vi "HFRR ADV v06.vi"() -> ()   [LabVIEW 2025] (continued)
            n1807 = for {
              N: w1967 -> [_]
              tunnel: w1981 -> [w2096]
              tunnel: w1980 -> [w2095]
              tunnel: [w2085] -> w1947 mode=indexing
              tunnel: [w2083] -> w1945 mode=indexing
              tunnel: [w2084] -> w1940 mode=indexing
              tunnel: w1966 -> [_]
              tunnel: [w2077] -> w1942 mode=indexing
              tunnel: [w2073] -> w1918 mode=indexing
              tunnel: [w2069] -> w1893 mode=indexing
              tunnel: [w2065] -> w1874 mode=indexing
              tunnel: [w2060] -> w1832 mode=indexing
              (unwired) TRUE ("line mode (F)")
              n1808 = Read from Text File "Read File"(file (use dialog)=w2096, error in=w2095) -> (text=w2061:string)  [unwired: 2 in, 3 out]
              n1809 = local write "String 7"(w2061) -> ()
              n1810 = String Subset(string=w2061, offset (0)=85, length (rest)=9 ("length (rest)")) -> (substring=w2064:string)
              n1811 = String Subset(string=w2061, offset (0)=35, length (rest)=9 ("length (rest)")) -> (substring=w2086:string)
              n1812 = String Subset(string=w2061, offset (0)=55, length (rest)=9 ("length (rest)")) -> (substring=w2072:string)
              n1813 = String Subset(string=w2061, offset (0)=25, length (rest)=9 ("length (rest)")) -> (substring=w2066:string)
              n1814 = String Subset(string=w2061, offset (0)=45, length (rest)=9 ("length (rest)")) -> (substring=w2074:string)
              n1815 = String Subset(string=w2061, offset (0)=0, length (rest)=14 ("length (rest)")) -> (substring=w2089:string)
              n1816 = String Subset(string=w2061, offset (0)=15, length (rest)=9 ("length (rest)")) -> (substring=w2092:string)
              n1817 = String Subset(string=w2061, offset (0)=65, length (rest)=9 ("length (rest)")) -> (substring=w2078:string)
              n1818 = Fract/Exp String To Number(string=w2064) -> (number=w2060:dbl)  [unwired: 3 in, 1 out]
              n1819 = Fract/Exp String To Number(string=w2086) -> (number=w2084:dbl)  [unwired: 3 in, 1 out]
              n1820 = Fract/Exp String To Number(string=w2072) -> (number=w2069:dbl)  [unwired: 3 in, 1 out]
              n1821 = Fract/Exp String To Number(string=w2066) -> (number=w2065:dbl)  [unwired: 3 in, 1 out]
              n1822 = Fract/Exp String To Number(string=w2074) -> (number=w2073:dbl)  [unwired: 3 in, 1 out]
              n1823 = Fract/Exp String To Number(string=w2089) -> (number=w2085:dbl)  [unwired: 3 in, 1 out]
              n1824 = Fract/Exp String To Number(string=w2092) -> (number=w2083:dbl)  [unwired: 3 in, 1 out]
              n1825 = Fract/Exp String To Number(string=w2078) -> (number=w2081:dbl)  [unwired: 3 in, 1 out]
              n1826 = Add(x=w2081, y=0.0) -> (x+y=w2077:dbl)
            }
            n1827 = for {
              N: w1969 -> [_]
              tunnel: w1976 -> [w2024]
              tunnel: w1975 -> [w2023]
              tunnel: [w2013] -> w1929 mode=indexing
              tunnel: [w2012] -> w1922 mode=indexing
              tunnel: w1966 -> [_]
              tunnel: [w2001] -> w1927 mode=indexing
              tunnel: [w2006] -> w1924 mode=indexing
              tunnel: [w2002] -> w1914 mode=indexing
              tunnel: [w1997] -> w1889 mode=indexing
              tunnel: [w1993] -> w1870 mode=indexing
              tunnel: [w1988] -> w1830 mode=indexing
              (unwired) 1.0 ("x")
              (unwired) TRUE ("line mode (F)")
              n1828 = Read from Text File "Read File"(file (use dialog)=w2024, error in=w2023) -> (text=w1989:string)  [unwired: 2 in, 3 out]
              n1829 = local write "String 12"(w1989) -> ()
              n1830 = String Subset(string=w1989, offset (0)=85, length (rest)=9 ("length (rest)")) -> (substring=w1991:string)
              n1831 = String Subset(string=w1989, offset (0)=35, length (rest)=9 ("length (rest)")) -> (substring=w2014:string)
              n1832 = String Subset(string=w1989, offset (0)=55, length (rest)=9 ("length (rest)")) -> (substring=w1999:string)
              n1833 = String Subset(string=w1989, offset (0)=25, length (rest)=9 ("length (rest)")) -> (substring=w1995:string)
              n1834 = String Subset(string=w1989, offset (0)=45, length (rest)=9 ("length (rest)")) -> (substring=w2004:string)
              n1835 = String Subset(string=w1989, offset (0)=15, length (rest)=9 ("length (rest)")) -> (substring=w2020:string)
              n1836 = String Subset(string=w1989, offset (0)=0, length (rest)=14 ("length (rest)")) -> (substring=w2017:string)
              n1837 = String Subset(string=w1989, offset (0)=65, length (rest)=9 ("length (rest)")) -> (substring=w2007:string)
              n1838 = Fract/Exp String To Number(string=w1991) -> (number=w1988:dbl)  [unwired: 3 in, 1 out]
              n1839 = Fract/Exp String To Number(string=w2014) -> (number=w2012:dbl)  [unwired: 3 in, 1 out]
              n1840 = Fract/Exp String To Number(string=w1999) -> (number=w1997:dbl)  [unwired: 3 in, 1 out]
              n1841 = Fract/Exp String To Number(string=w1995) -> (number=w1993:dbl)  [unwired: 3 in, 1 out]
              n1842 = Fract/Exp String To Number(string=w2004) -> (number=w2002:dbl)  [unwired: 3 in, 1 out]
              n1843 = Fract/Exp String To Number(string=w2020) -> (number=w2001:dbl)  [unwired: 3 in, 1 out]
              n1844 = Fract/Exp String To Number(string=w2017) -> (number=w2013:dbl)  [unwired: 3 in, 1 out]
              n1845 = Fract/Exp String To Number(string=w2007) -> (number=w2010:dbl)  [unwired: 3 in, 1 out]
              n1846 = Add(x=w2010, y=0.0) -> (x+y=w2006:dbl)
            }
            n1847 = Delete From Array(array=w1872, index=0) -> (array with subset deleted=w1845:dbl[])  [unwired: 1 in, 1 out]
            n1848 = Delete From Array(array=w1935, index=0) -> (array with subset deleted=w1908:dbl[])  [unwired: 1 in, 1 out]
            n1849 = Delete From Array(array=w1915, index=0) -> (array with subset deleted=w1903:dbl[])  [unwired: 1 in, 1 out]
            n1850 = Delete From Array(array=w1933, index=0) -> (array with subset deleted=w1934:dbl[])  [unwired: 1 in, 1 out]
            n1851 = call-poly <vilib>:"Mean.vi"("X"=w1845) -> ("mean"=→"КОФ2 4":dbl)  [unwired: 1 out]
            n1852 = call-poly <vilib>:"Mean.vi"("X"=w1908) -> ("mean"=→"КОФ3":dbl)  [unwired: 1 out]
            n1853 = call-poly <vilib>:"Mean.vi"("X"=w1903) -> ("mean"=→"CP3":dbl)  [unwired: 1 out]
            n1854 = Delete From Array(array=w1897, index=0) -> (array with subset deleted=w1824:dbl[])  [unwired: 1 in, 1 out]
            n1855 = Delete From Array(array=w1836, index=0) -> (array with subset deleted=w1823:dbl[])  [unwired: 1 in, 1 out]
            n1856 = Delete From Array(array=w1876, index=0) -> (array with subset deleted=w1847:dbl[])  [unwired: 1 in, 1 out]
            n1857 = Delete From Array(array=w1954, index=0) -> (array with subset deleted=w1909:dbl[])  [unwired: 1 in, 1 out]
            n1858 = Delete From Array(array=w1920, index=0) -> (array with subset deleted=w1905:dbl[])  [unwired: 1 in, 1 out]
            "array w/ subset deleted" <- w1905
            n1859 = Delete From Array(array=w1951, index=0) -> (array with subset deleted=w1952:dbl[])  [unwired: 1 in, 1 out]
            n1860 = call-poly <vilib>:"Mean.vi"("X"=w1847) -> ("mean"=→"КОФ2 2":dbl)  [unwired: 1 out]
            n1861 = call-poly <vilib>:"Mean.vi"("X"=w1909) -> ("mean"=→"КОФ1":dbl)  [unwired: 1 out]
            n1862 = Bundle "Bundle"(w1824, w1823) -> (w1829:cluster{dbl[], dbl[]})  [unwired: 1 in]
            n1863 = Bundle "Bundle"(w1824, w1952) -> (w1816:cluster{dbl[], dbl[]})  [unwired: 1 in]
            n1864 = Delete From Array(array=w1831, index=0) -> (array with subset deleted=w1819:dbl[])  [unwired: 1 in, 1 out]
            n1865 = Delete From Array(array=w1832, index=0) -> (array with subset deleted=w1821:dbl[])  [unwired: 1 in, 1 out]
            n1866 = Delete From Array(array=w1942, index=0) -> (array with subset deleted=w1943:dbl[])  [unwired: 1 in, 1 out]
            n1867 = Delete From Array(array=w1830, index=0) -> (array with subset deleted=w1817:dbl[])  [unwired: 1 in, 1 out]
            n1868 = Delete From Array(array=w1924, index=0) -> (array with subset deleted=w1925:dbl[])  [unwired: 1 in, 1 out]
            n1869 = Delete From Array(array=w1949, index=0) -> (array with subset deleted=w1855:dbl[])  [unwired: 1 in, 1 out]
            n1870 = Delete From Array(array=w1895, index=0) -> (array with subset deleted=w1851:dbl[])  [unwired: 1 in, 1 out]
            n1871 = Delete From Array(array=w1931, index=0) -> (array with subset deleted=w1853:dbl[])  [unwired: 1 in, 1 out]
            n1872 = Delete From Array(array=w1891, index=0) -> (array with subset deleted=w1849:dbl[])  [unwired: 1 in, 1 out]
            n1873 = Delete From Array(array=w1940, index=0) -> (array with subset deleted=w1854:dbl[])  [unwired: 1 in, 1 out]
            n1874 = Delete From Array(array=w1893, index=0) -> (array with subset deleted=w1850:dbl[])  [unwired: 1 in, 1 out]
            n1875 = Delete From Array(array=w1874, index=0) -> (array with subset deleted=w1846:dbl[])  [unwired: 1 in, 1 out]
            n1876 = Delete From Array(array=w1918, index=0) -> (array with subset deleted=w1904:dbl[])  [unwired: 1 in, 1 out]
            n1877 = Delete From Array(array=w1945, index=0) -> (array with subset deleted=w1906:dbl[])  [unwired: 1 in, 1 out]
            n1878 = Delete From Array(array=w1922, index=0) -> (array with subset deleted=w1852:dbl[])  [unwired: 1 in, 1 out]
            n1879 = Delete From Array(array=w1889, index=0) -> (array with subset deleted=w1848:dbl[])  [unwired: 1 in, 1 out]
            n1880 = Delete From Array(array=w1870, index=0) -> (array with subset deleted=w1844:dbl[])  [unwired: 1 in, 1 out]
            n1881 = Delete From Array(array=w1914, index=0) -> (array with subset deleted=w1902:dbl[])  [unwired: 1 in, 1 out]
            n1882 = Delete From Array(array=w1927, index=0) -> (array with subset deleted=w1907:dbl[])  [unwired: 1 in, 1 out]
            n1883 = Delete From Array(array=w1937, index=0) -> (array with subset deleted=w1820:dbl[])  [unwired: 1 in, 1 out]
            n1884 = Delete From Array(array=w1947, index=0) -> (array with subset deleted=w1822:dbl[])  [unwired: 1 in, 1 out]
            n1885 = Delete From Array(array=w1929, index=0) -> (array with subset deleted=w1818:dbl[])  [unwired: 1 in, 1 out]
            n1886 = Bundle "Bundle"(w1824, w1855) -> (w1842:cluster{dbl[], dbl[]})  [unwired: 1 in]
            n1887 = Bundle "Bundle"(w1824, w1909) -> (w1843:cluster{dbl[], dbl[]})  [unwired: 1 in]
            n1888 = Bundle "Bundle"(w1855, w1851) -> (w1857:cluster{dbl[], dbl[]})  [unwired: 1 in]
            n1889 = Bundle "Bundle"(w1820, w1819) -> (w1827:cluster{dbl[], dbl[]})  [unwired: 1 in]
            n1890 = Bundle "Bundle"(w1853, w1849) -> (w1859:cluster{dbl[], dbl[]})  [unwired: 1 in]
            n1891 = Bundle "Bundle"(w1820, w1853) -> (w1963:cluster{dbl[], dbl[]})  [unwired: 1 in]
            n1892 = Bundle "Bundle"(w1820, w1849) -> (w1887:cluster{dbl[], dbl[]})  [unwired: 1 in]
            n1893 = Bundle "Bundle"(w1820, w1908) -> (w1973:cluster{dbl[], dbl[]})  [unwired: 1 in]
            n1894 = Bundle "Bundle"(w1820, w1903) -> (w1911:cluster{dbl[], dbl[]})  [unwired: 1 in]
            n1895 = Bundle "Bundle"(w1820, w1934) -> (w1958:cluster{dbl[], dbl[]})  [unwired: 1 in]
            n1896 = Bundle "Bundle"(w1854, w1850) -> (w1858:cluster{dbl[], dbl[]})  [unwired: 1 in]
            n1897 = Bundle "Bundle"(w1822, w1821) -> (w1828:cluster{dbl[], dbl[]})  [unwired: 1 in]
            n1898 = Bundle "Bundle"(w1822, w1854) -> (w1965:cluster{dbl[], dbl[]})  [unwired: 1 in]
            n1899 = Bundle "Bundle"(w1822, w1850) -> (w1888:cluster{dbl[], dbl[]})  [unwired: 1 in]
            n1900 = Bundle "Bundle"(w1822, w1904) -> (w1912:cluster{dbl[], dbl[]})  [unwired: 1 in]
            n1901 = Bundle "Bundle"(w1822, w1906) -> (w1974:cluster{dbl[], dbl[]})  [unwired: 1 in]
            n1902 = Bundle "Bundle"(w1822, w1943) -> (w1956:cluster{dbl[], dbl[]})  [unwired: 1 in]
            n1903 = Bundle "Bundle"(w1852, w1848) -> (w1860:cluster{dbl[], dbl[]})  [unwired: 1 in]
            n1904 = Bundle "Bundle"(w1818, w1817) -> (w1826:cluster{dbl[], dbl[]})  [unwired: 1 in]
            n1905 = Bundle "Bundle"(w1818, w1852) -> (w1964:cluster{dbl[], dbl[]})  [unwired: 1 in]
            n1906 = Bundle "Bundle"(w1818, w1848) -> (w1886:cluster{dbl[], dbl[]})  [unwired: 1 in]
            n1907 = Bundle "Bundle"(w1818, w1902) -> (w1910:cluster{dbl[], dbl[]})  [unwired: 1 in]
            n1908 = Bundle "Bundle"(w1818, w1907) -> (w1972:cluster{dbl[], dbl[]})  [unwired: 1 in]
            n1909 = Bundle "Bundle"(w1818, w1925) -> (w1957:cluster{dbl[], dbl[]})  [unwired: 1 in]
            n1910 = call-poly <vilib>:"Mean.vi"("X"=w1905) -> ("mean"=→"CP1":dbl)  [unwired: 1 out]
            n1911 = call-poly <vilib>:"Mean.vi"("X"=w1846) -> ("mean"=→"КОФ2 3":dbl)  [unwired: 1 out]
            n1912 = call-poly <vilib>:"Mean.vi"("X"=w1904) -> ("mean"=→"CP2":dbl)  [unwired: 1 out]
            n1913 = call-poly <vilib>:"Mean.vi"("X"=w1906) -> ("mean"=→"КОФ2":dbl)  [unwired: 1 out]
            n1914 = call-poly <vilib>:"Mean.vi"("X"=w1844) -> ("mean"=→"КОФ2 5":dbl)  [unwired: 1 out]
            n1915 = call-poly <vilib>:"Mean.vi"("X"=w1902) -> ("mean"=→"CP4":dbl)  [unwired: 1 out]
            n1916 = call-poly <vilib>:"Mean.vi"("X"=w1907) -> ("mean"=→"КОФ4":dbl)  [unwired: 1 out]
            n1917 = Bundle "Bundle"(w1824, w1851) -> (w1815:cluster{dbl[], dbl[]})  [unwired: 1 in]
            n1918 = Bundle "Bundle"(w1824, w1905) -> (w1838:cluster{dbl[], dbl[]})  [unwired: 1 in]
            n1919 = Build Array "Build Array"(w1815, w1838) -> (w1841:cluster{dbl[], dbl[]}[])
            "XY Graph 17" <- w1841
            n1920 = Build Array "Build Array"(w1829, w1828, w1827, w1826) -> (→"Frequency ( Hz )":cluster{dbl[], dbl[]}[])
            n1921 = Build Array "Build Array"(w1857, w1858, w1859, w1860) -> (→"Air Temp ( °C ) vs Humidity ( % RH )":cluster{dbl[], dbl[]}[])
            n1922 = Build Array "Build Array"(w1842, w1965, w1963, w1964) -> (→"Air Temperature  ( °C )":cluster{dbl[], dbl[]}[])
            n1923 = Build Array "Build Array"(w1815, w1888, w1887, w1886) -> (→"Humidity ( %RH )":cluster{dbl[], dbl[]}[])
            n1924 = Build Array "Build Array"(w1843, w1974, w1973, w1972) -> (→"Coefficient Of Friction":cluster{dbl[], dbl[]}[])
            n1925 = Build Array "Build Array"(w1838, w1912, w1911, w1910) -> (→"Sample Temperature ( °C )":cluster{dbl[], dbl[]}[])
            n1926 = Build Array "Build Array"(w1816, w1956, w1958, w1957) -> (→"XY Graph 13":cluster{dbl[], dbl[]}[])
            n1927 = Bundle "Bundle"(w1824, w1847) -> (w1869:cluster{dbl[], dbl[]})  [unwired: 1 in]
            n1928 = Bundle "Bundle"(w1820, w1845) -> (w1867:cluster{dbl[], dbl[]})  [unwired: 1 in]
            n1929 = Bundle "Bundle"(w1822, w1846) -> (w1868:cluster{dbl[], dbl[]})  [unwired: 1 in]
            n1930 = Bundle "Bundle"(w1818, w1844) -> (w1866:cluster{dbl[], dbl[]})  [unwired: 1 in]
            n1931 = Build Array "Build Array"(w1869, w1868, w1867, w1866) -> (→"Stroke ( mm )":cluster{dbl[], dbl[]}[])
            n1932 = local write "XY Graph 16"(w1841) -> ()
          }
          frame #2 {
          }
          frame #3 {
            n1933 = local write "Numeric 8"(0 ("Numeric 8")) -> ()
            n1934 = local write "Numeric 11"(0 ("Numeric 11")) -> ()
            n1935 = local write "Numeric 12"(0 ("Numeric 12")) -> ()
            n1936 = local write "Numeric 13"(0 ("Numeric 13")) -> ()
            n1937 = property on="OPEN" class="Bool (strict)"("Visible"=TRUE) -> ()  [unwired: 2 in, 2 out]
            n1938 = local read "String Control 2"() -> (w2141:string)
            n1939 = local read "String Control 4"() -> (w2140:string)
            n1940 = local read "String Control 6"() -> (w2139:string)
            n1941 = local read "String Control 8"() -> (w2138:string)
            n1942 = Match Pattern(string=w2141, regular expression="Samples / cycle :- ") -> (after substring=w2155:string)  [unwired: 1 in, 3 out]
            n1943 = Match Pattern(string=w2141, regular expression="Frequency :- ") -> (after substring=w2174:string)  [unwired: 1 in, 3 out]
            n1944 = Match Pattern(string=w2140, regular expression="Samples / cycle :- ") -> (after substring=w2151:string)  [unwired: 1 in, 3 out]
            n1945 = Match Pattern(string=w2140, regular expression="Frequency :- ") -> (after substring=w2169:string)  [unwired: 1 in, 3 out]
            n1946 = Match Pattern(string=w2139, regular expression="Samples / cycle :- ") -> (after substring=w2147:string)  [unwired: 1 in, 3 out]
            n1947 = Match Pattern(string=w2139, regular expression="Frequency :- ") -> (after substring=w2164:string)  [unwired: 1 in, 3 out]
            n1948 = Match Pattern(string=w2138, regular expression="Samples / cycle :- ") -> (after substring=w2143:string)  [unwired: 1 in, 3 out]
            n1949 = Match Pattern(string=w2138, regular expression="Frequency :- ") -> (after substring=w2159:string)  [unwired: 1 in, 3 out]
            n1950 = String Subset(string=w2155, length (rest)=6 ("length (rest)")) -> (substring=w2157:string)  [unwired: 1 in]
            n1951 = String Subset(string=w2174, length (rest)=9 ("length (rest)")) -> (substring=w2176:string)  [unwired: 1 in]
            n1952 = String Subset(string=w2151, length (rest)=6 ("length (rest)")) -> (substring=w2153:string)  [unwired: 1 in]
            n1953 = String Subset(string=w2169, length (rest)=9 ("length (rest)")) -> (substring=w2171:string)  [unwired: 1 in]
            n1954 = String Subset(string=w2147, length (rest)=6 ("length (rest)")) -> (substring=w2149:string)  [unwired: 1 in]
            n1955 = String Subset(string=w2164, length (rest)=9 ("length (rest)")) -> (substring=w2166:string)  [unwired: 1 in]
            n1956 = String Subset(string=w2143, length (rest)=6 ("length (rest)")) -> (substring=w2145:string)  [unwired: 1 in]
            n1957 = String Subset(string=w2159, length (rest)=9 ("length (rest)")) -> (substring=w2161:string)  [unwired: 1 in]
            n1958 = Fract/Exp String To Number(string=w2157) -> (number=w2137:dbl)  [unwired: 3 in, 1 out]
            n1959 = Fract/Exp String To Number(string=w2176) -> (number=w2177:dbl)  [unwired: 3 in, 1 out]
            n1960 = Fract/Exp String To Number(string=w2153) -> (number=w2136:dbl)  [unwired: 3 in, 1 out]
            n1961 = Fract/Exp String To Number(string=w2171) -> (number=w2172:dbl)  [unwired: 3 in, 1 out]
            n1962 = Fract/Exp String To Number(string=w2149) -> (number=w2135:dbl)  [unwired: 3 in, 1 out]
            n1963 = Fract/Exp String To Number(string=w2166) -> (number=w2167:dbl)  [unwired: 3 in, 1 out]
            n1964 = Fract/Exp String To Number(string=w2145) -> (number=w2134:dbl)  [unwired: 3 in, 1 out]
            n1965 = Fract/Exp String To Number(string=w2161) -> (number=w2162:dbl)  [unwired: 3 in, 1 out]
            n1966 = local write "sample1"(w2137) -> ()
            n1967 = local write "freq1"(w2177) -> ()
            n1968 = local write "sample2"(w2136) -> ()
            n1969 = local write "freq2"(w2172) -> ()
            n1970 = local write "sample3"(w2135) -> ()
            n1971 = local write "freq3"(w2167) -> ()
            n1972 = local write "sample4"(w2134) -> ()
            n1973 = local write "freq 4"(w2162) -> ()
          }
        }
      }
    }
    n1974 = case shown="True" w1626 {
      selector: w1626 -> [_ w1754]
      frame False {
      }
      frame True {
        n1975 = Not(x=w1754) -> (.not. x?=w1750:bool)
        n1976 = local write "service 3"(w1750) -> ()
        n1977 = local write "OPEN 6"(w1750) -> ()
        n1978 = call <vilib>:"System Exec.vi"("wait until completion? (T)"=TRUE, "command line"="C:\\LAB-IQ\\Scar View.exe") -> ("error out"=→"error out 5":errorcluster)  [unwired: 6 in, 3 out]
      }
    }
    n1979 = case shown="\"Acquire\", Default" w1637 {
      frame "Acquire", Default {
        w2650 = 0.2 ("y")
        w2655 = 1.0 ("y")
        w2656 = 0.8 ("y")
        # "Elapsed time\ncof\nstroke\nAir temp\nTemp\nHumidity"
        n1980 = disable-structure shown="Disabled" {
          frame Disabled {
            n1981 = local read "Flag"() -> (w2673:dbl)
            n1982 = local read "RUN"() -> (w2670:bool)
            n1983 = Not(x=w2670) -> (.not. x?=w2669:bool)
            n1984 = Equal?(x=w2673, y=10.0) -> (x = y?=w2671:bool)
            n1985 = And(x=w2671, y=w2669) -> (x .and. y?=w2668:bool)
            n1986 = case shown="True" w2668 {
              frame False {
              }
              frame True {
                w2674 = FALSE ("Heater Button")
                n1987 = local write "Humidity"(w2674) -> ()
                n1988 = local write "Heater Button"(w2674) -> ()
              }
            }
          }
          frame Enabled {
          }
        }
        n1989 = disable-structure shown="Disabled" {
          frame Disabled {
            n1990 = case shown="True" {
              selector: _ -> [_ _]
              frame False {
              }
              frame True {
                w2765 = TRUE ("Heater")
                n1991 = local write "Humidity"(w2765) -> ()
                n1992 = local write "Heater Button"(w2765) -> ()
                n1993 = local read "TEST STANDARD"() -> (w2768:T3)
                n1994 = local read "TEST STANDARD"() -> (w2763:T3)
                n1995 = Equal?(x=w2768, y=enum16{"ASTM D6079", "ISO 12156", "Custom"}."ISO 12156" ("Test Standard")) -> (x = y?=w2766:bool)
                n1996 = Equal?(x=w2763, y=enum16{"ASTM D6079", "ISO 12156", "Custom"}."ASTM D6079" ("Test Standard")) -> (x = y?=w2762:bool)
                n1997 = case shown="True" w2766 {
                  frame False {
                  }
                  frame True {
                    n1998 = local write "Heater"(TRUE ("Heater")) -> ()
                    n1999 = local write "airtempflg"(FALSE ("airtempflg")) -> ()
                  }
                }
                n2000 = case shown="True" w2762 {
                  frame False {
                  }
                  frame True {
                    n2001 = local write "Heater"(FALSE ("Heater")) -> ()
                    n2002 = local write "airtempflg"(TRUE ("airtempflg")) -> ()
                  }
                }
              }
            }
          }
          frame Enabled {
          }
        }
        n2003 = stacked-sequence {
          frame #0 {
            n2004 = case shown="True" "RST FF" {
              frame False {
              }
              frame True {
                w2831 = 0.0 ("X Scale.Range:Maximum")
                n2005 = property on="Frictional Force ( N )" class="WFChart (strict)"("XScale.Maximum"=600.0 ("X Scale.Range:Maximum"), "XScale.Minimum"=w2831, "YScale.Maximum"=10.0 ("Y Scale.Range:Maximum"), "YScale.Minimum"=w2831) -> ()  [unwired: 2 in, 2 out]
              }
            }
          }
          frame #1 {
            n2006 = case shown="True" "RST TEMP" {
              frame False {
              }
              frame True {
                n2007 = property on="Temperature ( Deg C )" class="WFChart (strict)"("XScale.Minimum"=0.0 ("X Scale.Range:Minimum"), "XScale.Maximum"=600.0 ("X Scale.Range:Maximum"), "YScale.Minimum"=0.0 ("Y Scale.Range:Minimum"), "YScale.Maximum"=100.0 ("Y Scale.Range:Maximum")) -> ()  [unwired: 2 in, 2 out]
              }
            }
          }
          frame #2 {
            n2008 = case shown="True" "RSTCOF" {
              frame False {
              }
              frame True {
                n2009 = property on="Coefficient of Friction" class="WFChart (strict)"("XScale.Minimum"=0.0 ("X Scale.Range:Minimum"), "XScale.Maximum"=600.0 ("X Scale.Range:Maximum"), "YScale.Maximum"=1.0 ("X Scale.Range:Minimum"), "YScale.Minimum"=0.0 ("X Scale.Range:Minimum")) -> ()  [unwired: 2 in, 2 out]
              }
            }
          }
          frame #3 {
            n2010 = case shown="True" "RSTCOF 2" {
              frame False {
              }
              frame True {
                (unwired) 100.0 ("Y Scale.Range:Maximum")
                (unwired) 0.0 ("Y Scale.Range:Minimum")
                (unwired) 600.0 ("X Scale.Range:Maximum")
                (unwired) 0.0 ("X Scale.Range:Minimum")
              }
            }
          }
          frame #4 {
            n2011 = case shown="True" "RSTCOF 3" {
              frame False {
              }
              frame True {
                n2012 = property on="Electrical Contact Resistance ( % )" class="WFChart (strict)"("XScale.Minimum"=0.0 ("X Scale.Range:Minimum"), "XScale.Maximum"=600.0 ("X Scale.Range:Maximum"), "YScale.Minimum"=0.0 ("Y Scale.Range:Minimum"), "YScale.Maximum"=100.0 ("Y Scale.Range:Maximum")) -> ()  [unwired: 2 in, 2 out]
              }
            }
          }
        }
        n2013 = disable-structure shown="Disabled" {
          frame Disabled {
            n2014 = case shown="True" {
              selector: _ -> [_ _]
              frame False {
              }
              frame True {
                n2015 = local read "zflag 2"() -> (w2732:dbl)
                n2016 = local read "yflag"() -> (w2734:dbl)
                n2017 = Equal?(x=w2734, y=2.0 ("tflag")) -> (x = y?=w2736:bool)
                n2018 = Equal?(x=w2732, y=3.0 ("tflag")) -> (x = y?=w2735:bool)
                n2019 = And(x=w2736, y=w2735) -> (x .and. y?=w2730:bool)
                n2020 = case shown="True" w2730 {
                  frame False {
                  }
                  frame True {
                    w2761 = 0.0 ("zflag")
                    n2021 = local write "zflag"(w2761) -> ()
                    n2022 = local write "zflag 2"(w2761) -> ()
                    n2023 = Delete(path (use dialog)=path "C:/LAB-IQ-NXT/WO 2449 TT.sig" ("file path (dialog if empty)")) -> (deleted path=w2760:path)  [unwired: 4 in, 2 out]
                    n2024 = Delete(path (use dialog)=path "C:/LAB-IQ-NXT/WO 2449 TRH.sig" ("file path (dialog if empty)")) -> (deleted path=w2755:path)  [unwired: 4 in, 2 out]
                    n2025 = local read "SEN.RUN HRS"() -> (w2747:dbl)
                    n2026 = local read "SENSOR TIME"() -> (w2745:dbl)
                    n2027 = call <vilib>:"compatOverwrite.vi"("overwrite (F)"=TRUE) -> ("overwrite?"=w2737:T27)
                    n2028 = call <vilib>:"compatOverwrite.vi"("overwrite (F)"=TRUE) -> ("overwrite?"=w2741:T27)
                    n2029 = local read "Total No. of Tests"() -> (w2748:dbl)
                    n2030 = Add(x=w2745, y=w2747) -> (x+y=w2746:dbl)
                    "SEN.RUN HRS" <- w2746
                    n2031 = Open/Create/Replace File(file path (use dialog)=w2760, operation (0:open)=w2737) -> (refnum out=w2738:refnum<file>, error out=w2739:errorcluster)  [unwired: 4 in, 1 out]
                    n2032 = Open/Create/Replace File(file path (use dialog)=w2755, operation (0:open)=w2741) -> (refnum out=w2742:refnum<file>, error out=w2743:errorcluster)  [unwired: 4 in, 1 out]
                    n2033 = Deny Access(4:w2739, 6:T24."deny none" ("deny mode (2)"), 7:w2738) -> (3:w2759:refnum<file>)  [unwired: 1 out]
                    n2034 = Deny Access(4:w2743, 6:T24."deny none" ("deny mode (2)"), 7:w2742) -> (3:w2751:refnum<file>)  [unwired: 1 out]
                    n2035 = Number To Decimal String(number=w2748) -> (decimal integer string=w2756:string)  [unwired: 1 in]
                    n2036 = Number To Decimal String(number=w2746) -> (decimal integer string=w2752:string)  [unwired: 1 in]
                    n2037 = Write to Binary File(file (use dialog)=w2759, data=w2756, 5:FALSE ("prepend array or string size? (T)")) -> ()  [unwired: 3 in, 3 out]
                    n2038 = Write to Binary File(file (use dialog)=w2751, data=w2752, 5:FALSE ("prepend array or string size? (T)")) -> ()  [unwired: 3 in, 3 out]
                  }
                }
              }
            }
          }
          frame Enabled {
          }
        }
        n2039 = local read "RUN"() -> (w2659:bool)
        n2040 = local read "run replace"() -> (w2663:bool)
        n2041 = local read "run replace"() -> (w2662:bool)
        n2042 = case shown="True" w2659 {
          frame False {
            n2043 = local write "run replace"(FALSE ("run replace")) -> ()
          }
          frame True {
            "run replace" <- TRUE ("run replace")
          }
        }
        n2044 = local read "RUN"() -> (w2667:bool)
        n2045 = local read "Set Temp"() -> (w2629:dbl)
        n2046 = local read "SetTemp"() -> (w2631:dbl)
        n2047 = case shown="False" w2667 {
          tunnel: [FALSE ("TEST RUNNING") TRUE ("TEST RUNNING")] -> w2666
          frame False {
            w2850 = 0.0 ("Flag")
            n2048 = local write "Elapsed time"(0.0 ("elapsedtime")) -> ()
            n2049 = local write "Time Remaining"(w2850) -> ()
            n2050 = local write "Flag"(w2850) -> ()
            n2051 = local write "Remaining Time"(w2850) -> ()
          }
          frame True {
            n2052 = local write "Flag"(10.0 ("Flag")) -> ()
          }
        }
        n2053 = case shown="False" w2663 {
          frame False {
            n2054 = local read "zflag"() -> (→"zflag 2":dbl)
            n2055 = local write "yflag"(2.0 ("tflag")) -> ()
            n2056 = local write "FLAG 4"(0.0 ("FLAG")) -> ()
          }
          frame True {
            n2057 = local write "yflag"(1.0 ("tflag")) -> ()
            n2058 = local write "zflag"(3.0 ("zflag")) -> ()
          }
        }
        n2059 = local read "acq 2"() -> (w2661:bool)
        n2060 = local read "AIR TEMP"() -> (w2624:dbl)
        n2061 = local read "Amb temp"() -> (w2628:dbl)
        n2062 = case shown="True" "Save & Continue" {
          frame False {
          }
          frame True {
            "acq 2" <- TRUE ("acq 2")
          }
        }
        n2063 = local read "Set Rh"() -> (w2630:dbl)
        n2064 = Add(x=w2631, y=w2656) -> (x+y=w2657:dbl)
        n2065 = Subtract(x=w2631, y=w2656) -> (x-y=w2658:dbl)
        n2066 = Add(x=w2629, y=w2650) -> (x+y=w2651:dbl)
        n2067 = Subtract(x=w2629, y=w2650) -> (x-y=w2652:dbl)
        n2068 = And(x=w2661, y=w2662) -> (x .and. y?=w2660:bool)
        n2069 = Greater Or Equal?(x=w2624, y=15.0) -> (x >= y?=w2625:bool)
        "powstat" <- w2625
        n2070 = local read "Humidity ( %RH )"() -> (w2627:dbl)
        n2071 = case shown="True" "Save & Continue" {
          frame False {
          }
          frame True {
            n2072 = while {
              tunnel: "0123456789abcdefghijklmnopqrstuvwxyzABCDEFGHIJKLMNOPQRSTUVWXYZ" ("string 2") -> [w2821]
              shift-right: [w2819] -> w2814
              shift-left: "" -> [w2818]
              i -> [w2828]
              stop <- w2827 stop-if-true
              n2073 = Random Number (0-1)() -> (number: 0 to 1=w2822:dbl)
              n2074 = Multiply(x=w2822, y=62.0) -> (x*y=w2824:dbl)
              n2075 = Decrement(x="Length") -> (x-1=w2817:i16)
              n2076 = To Word Integer(number=w2824) -> (16bit integer=w2825:i16)
              n2077 = String Subset(string=w2821, offset (0)=w2825, length (rest)=1 ("length (rest)")) -> (substring=w2820:string)
              n2078 = Greater Or Equal?(x=w2828, y=w2817) -> (x >= y?=w2827:bool)
              n2079 = Concatenate Strings(w2820, w2818) -> (w2819:string)
            }
            n2080 = local write "UUID"(w2814) -> ()
          }
        }
        n2081 = In Range and Coerce(upper limit=w2657, x=w2628, lower limit=w2658) -> (In Range?=w2647:bool)  [unwired: 1 out]
        n2082 = Add(x=w2630, y=w2655) -> (x+y=w2654:dbl)
        n2083 = Subtract(x=w2630, y=w2655) -> (x-y=w2653:dbl)
        n2084 = local read "TEMP"() -> (w2626:dbl)
        n2085 = case shown="True" "Save & Continue" {
          frame False {
          }
          frame True {
            n2086 = local read "Operator ID"() -> (w3130:string)
            n2087 = local read "FILE"() -> (w3136:string)
            n2088 = String Length(string=w3136) -> (length=w3134:i32)
            n2089 = String Length(string=w3130) -> (length=w3131:i32)
            n2090 = Greater?(x=w3134, y=0) -> (0:w3133:bool)
            n2091 = Greater?(x=w3131, y=0) -> (0:w3129:bool)
            n2092 = And(x=w3133, y=w3129) -> (x .and. y?=w3128:bool)
            n2093 = case shown="True" w3128 {
              frame False {
                n2094 = stacked-sequence {
                  frame #0 {
                    n2095 = One Button Dialog(message="Please Enter a File Name and Operator ID to save data !", button name ("OK")="Ok") -> ()  [unwired: 1 out]
                  }
                  frame #1 {
                    n2096 = local write "Save & Continue"(FALSE ("OK Button")) -> ()
                  }
                }
                n2097 = local write "Save & Continue"(FALSE ("OK Button")) -> ()
              }
              frame True {
                n2098 = stacked-sequence {
                  frame #0 {
                    n2099 = local read "FILE"() -> (w3142:string)
                    n2100 = call "file check.vi"("file name in"=w3142) -> ("file name out"=w3141:string)  [unwired: 9 in, 1 out]
                    n2101 = call <vilib>:"Application Directory.vi"() -> ("Application Directory"=w3152:path)
                    n2102 = Build Path(base path=w3152, name or relative path="data") -> (appended path=w3151:path)
                    n2103 = call <vilib>:"Trim Whitespace.vi"("string"=w3141) -> ("trimmed string"=w3149:string)  [unwired: 1 in]
                    n2104 = call <vilib>:"Trim Whitespace.vi"("string"=w3141) -> ("trimmed string"=w3150:string)  [unwired: 1 in]
                    n2105 = List Folder(path=w3151) -> (folder names=w3147:string[])  [unwired: 3 in, 3 out]
                    n2106 = Match Pattern(string=w3149, regular expression="_(") -> (before substring=w3146:string)  [unwired: 1 in, 3 out]
                    n2107 = for {
                      tunnel: w3147 -> [w3161] mode=indexing
                      tunnel: w3146 -> [w3159]
                      shift-right: [w3157] -> w3144
                      shift-left: bool[] [] -> [w3158]
                      n2108 = Match Pattern(string=w3161, regular expression="_(") -> (before substring=w3160:string)  [unwired: 1 in, 3 out]
                      n2109 = Equal?(x=w3160, y=w3159) -> (x = y?=w3156:bool)
                      n2110 = case shown="True" w3156 {
                        tunnel: w3156 -> [_ w3164]
                        tunnel: w3158 -> [w3163 w3166]
                        tunnel: [w3163 w3165] -> w3157
                        frame False {
                        }
                        frame True {
                          n2111 = Insert Into Array(array=w3166, new element=w3164) -> (w3165:bool[])  [unwired: 1 in]
                        }
                      }
                    }
                    n2112 = Equal?(x=w3147, y=w3146) -> (x = y?=w3155:bool[])
                    n2113 = Or Array Elements(Boolean array=w3155) -> (logical OR=w3154:bool)
                    n2114 = Array Size(array=w3144) -> (size(s)=w3143:i32)
                    n2115 = case shown="True" w3154 {
                      tunnel: w3150 -> [_ w3174]
                      tunnel: w3143 -> [_ w3167]
                      frame False {
                      }
                      frame True {
                        n2116 = Number To Decimal String(number=w3167) -> (decimal integer string=w3170:string)  [unwired: 1 in]
                        n2117 = Search/Split String(string=w3174, search string/char (-)="_(" ("regular expression")) -> (substring before match=w3172:string)  [unwired: 1 in, 2 out]
                        n2118 = Concatenate Strings(w3172, "_(" ("regular expression"), w3170, ")" ("regular expression")) -> (w3168:string)
                        n2119 = local write "FILE"(w3168) -> ()
                      }
                    }
                  }
                  frame #1 {
                    w3176 = 0.0
                    w3189 = cluster{"y":dbl, dbl, "y":dbl}[] [] ("History Data")
                    w3190 = FALSE ("Heater Button")
                    (unwired) ")!" ("string")
                    (unwired) ")" ("string")
                    w3188 = dbl[] [] ("History Data")
                    w3194 = "\r"
                    # "C:\\WinDucom\\Data\\"
                    # "C:\\LAB-IQ-NXT\\data"
                    n2120 = local write "Humidity ( %RH )"(w3176) -> ()
                    n2121 = local write "Frequency ( Hz )"(w3176) -> ()
                    n2122 = local write "Stroke 3"(w3176) -> ()
                    n2123 = local write "speedop"(0.0 ("PIDclk 2")) -> ()
                    n2124 = local write "Set Temp 2"(65.0 ("Set Temp 2")) -> ()
                    n2125 = local write "AIR TEMP"(w3176) -> ()
                    n2126 = local write "clk"(0.0 ("clk")) -> ()
                    n2127 = local write "Stroke 4"(w3176) -> ()
                    n2128 = local write "COF 2"(w3176) -> ()
                    n2129 = local write "TEMP"(w3176) -> ()
                    n2130 = local write "ecr 3"(w3176) -> ()
                    n2131 = local write "FF 3"(w3176) -> ()
                    n2132 = local write "FF 2"(w3176) -> ()
                    n2133 = property on="Humidity ( %RH )" class="WFChart (strict)"("History Data"=w3188) -> ()  [unwired: 2 in, 2 out]
                    n2134 = property on="Coefficient of Friction" class="WFChart (strict)"("History Data"=w3188) -> ()  [unwired: 2 in, 2 out]
                    n2135 = property on="Coefficient of Friction" class="WFChart (strict)"("History Data"=w3188) -> ()  [unwired: 2 in, 2 out]
                    n2136 = property on="Frictional Force ( N )" class="WFChart (strict)"("History Data"=w3188) -> ()  [unwired: 2 in, 2 out]
                    n2137 = property on="Electrical Contact Resistance ( % )" class="WFChart (strict)"("History Data"=w3188) -> ()  [unwired: 2 in, 2 out]
                    n2138 = property on="Electrical Contact Resistance ( % )" class="WFChart (strict)"("History Data"=w3188) -> ()  [unwired: 2 in, 2 out]
                    n2139 = property on="Temperature ( Deg C )" class="WFChart (strict)"("History Data"=w3188) -> ()  [unwired: 2 in, 2 out]
                    n2140 = property on="Frictional Force ( N )" class="WFChart (strict)"("History Data"=w3188) -> ()  [unwired: 2 in, 2 out]
                    n2141 = property on="Coefficient of Friction" class="WFChart (strict)"("History Data"=w3188) -> ()  [unwired: 2 in, 2 out]
                    n2142 = property on="Frictional Force ( N )" class="WFChart (strict)"("History Data"=w3188) -> ()  [unwired: 2 in, 2 out]
                    n2143 = property on="Electrical Contact Resistance ( % )" class="WFChart (strict)"("History Data"=w3188) -> ()  [unwired: 2 in, 2 out]
                    n2144 = property on="Temperature ( Deg C )" class="WFChart (strict)"("History Data"=w3188) -> ()  [unwired: 2 in, 2 out]
                    n2145 = property on="Humidity ( %RH )" class="WFChart (strict)"("History Data"=w3188) -> ()  [unwired: 2 in, 2 out]
                    n2146 = property on="Stroke ( mm )" class="WFChart (strict)"("History Data"=w3189) -> ()  [unwired: 2 in, 2 out]
                    n2147 = property on="Stroke ( mm )" class="WFChart (strict)"("History Data"=w3189) -> ()  [unwired: 2 in, 2 out]
                    n2148 = local write "Humidity"(w3190) -> ()
                    n2149 = local write "Heater Button"(w3190) -> ()
                    n2150 = local read "FILE"() -> (w3184:string)
                    n2151 = disable-structure shown="Enabled" {
                      disable-tunnel: [w3229 _] -> w3175
                      frame Enabled {
                        n2152 = local read "NORMAL LOAD"() -> (w3229:dbl)
                      }
                      frame Disabled {
                      }
                    }
                    n2153 = call "file check.vi"("file name in"=w3184) -> ("error out"=w3187:errorcluster, "file name out"=w3181:string)  [unwired: 9 in]
                    n2154 = call "FILE PATH CREATION.vi"("error in"=w3187, "FILE NAME :"=w3181) -> ("FILE OUT"=w3180:path)  [unwired: 8 in, 1 out]
                    n2155 = Concatenate Strings(w3181, ".dgf" ("Substring")) -> (w3186:string)
                    n2156 = Concatenate Strings(w3181, ".duf" ("Substring")) -> (w3182:string)
                    n2157 = Multiply(x=w3175, y=1.0) -> (x*y=w3208:dbl)
                    n2158 = Build Path(base path=w3180, name or relative path=w3186) -> (appended path=w3179:path)
                    n2159 = Build Path(base path=w3180, name or relative path=w3182) -> (appended path=w3178:path)
                    n2160 = Number To Fractional String(number=w3208, width (-)=i16 5, precision (6)=i16 2) -> (F-format string=w3216:string)  [unwired: 1 in]
                    n2161 = local read "Fuel Discription :"() -> (w3204:string)
                    n2162 = local read "Batch Ref Num :"() -> (w3192:string)
                    n2163 = Get Date/Time String(date format (0)=enum16{"short", "long", "abbreviated"}."short") -> (date string=w3227:string, time string=w3224:string)  [unwired: 2 in]
                    n2164 = local read "Remarks :"() -> (w3203:string)
                    n2165 = Concatenate Strings("Load :- " ("Substring"), w3216, " grams ," ("Substring")) -> (w3215:string)
                    n2166 = local read "String 41"() -> (w3195:string)
                    n2167 = Concatenate Strings(w3204) -> (w3205:string)
                    n2168 = Concatenate Strings(w3192) -> (w3191:string)
                    n2169 = Concatenate Strings("tested by") -> (w3199:string)
                    n2170 = Concatenate Strings("(" ("Substring"), w3227, ")" ("Substring"), w3224) -> (w3197:string)
                    "concatenated string" <- w3197
                    n2171 = Concatenate Strings(w3203, "," ("string")) -> (w3202:string)
                    n2172 = Concatenate Strings("  TIME;      COF;       STROKE;     AIR TEMP;  TEMP;  HUMIDITY;  ECR; PID-OUT; FREQUENCY" ("Substring"), "\r") -> (w3211:string)
                    n2173 = Concatenate Strings(w3195, w3194, "Fuel Discription :-" ("Substring"), w3205, w3194, w3215, w3194, "Batch Ref Num :-" ("Substring"), w3191, w3194, " Remarks :- " ("Substring"), w3202, w3194, " Date :- " ("Substring"), w3197, w3194, "Tested By :-" ("Substring"), w3199) -> (w3209:string)
                    "REMARKS" <- w3209
                    n2174 = call <vilib>:"Write Characters To File.vi"("append to file? (new file:F)"=FALSE, "character string"=w3211, "file path (dialog if empty)"=w3179) -> ()  [unwired: 2 in, 1 out]
                    n2175 = call <vilib>:"Write Characters To File.vi"("append to file? (new file:F)"=FALSE, "character string"=w3209, "file path (dialog if empty)"=w3178) -> ()  [unwired: 2 in, 1 out]
                  }
                  frame #2 {
                    n2176 = local write "Cycles elapsed"(0 ("Cycles elapsed")) -> ()
                    n2177 = local write "cyclecount"(0 ("cyclecount")) -> ()
                    n2178 = local write "Save & Continue"(FALSE ("OK")) -> ()
                    n2179 = local write "autostrtflg"(TRUE ("autostrtflg")) -> ()
                    n2180 = local write "Save"(FALSE ("Save")) -> ()
                    n2181 = Get Date/Time In Seconds() -> (seconds since 1Jan1904=w3234:timestamp)
                    n2182 = To Double Precision Float(number=w3234) -> (double precision float=w3233:dbl)
                    n2183 = local write "acq timer"(w3233) -> ()
                    n2184 = One Button Dialog(message="Please ensure sample is mounted properly and machine is ready in all aspects for testing !", button name ("OK")="Ok") -> ()  [unwired: 1 out]
                  }
                  frame #3 {
                    n2185 = stacked-sequence {
                      frame #0 {
                        n2186 = local write "Main Dashboard Buttons"(T1."Dashboard" ("Main Dashboard Buttons")) -> ()
                        n2187 = local write "Main Tab"(T2."Acquire" ("Main Tab")) -> ()
                      }
                      frame #1 {
                        n2188 = local write "EVENT LOG"("" ("EVENT LOG")) -> ()
                      }
                      frame #2 {
                        n2189 = Wait (ms)(milliseconds to wait=u32 50) -> ()  [unwired: 1 out]
                      }
                      frame #3 {
                        n2190 = disable-structure shown="Disabled" {
                          frame Disabled {
                            n2191 = local read "EVENT LOG"() -> (w3246:string)
                            n2192 = call "Event Log.vi"("Content"="Test Details", "EVENT LOG"=w3246) -> ("EVENT LOG"=w3245:string)  [unwired: 8 in, 1 out]
                            n2193 = local write "EVENT LOG"(w3245) -> ()
                          }
                          frame Enabled {
                          }
                        }
                      }
                      frame #4 {
                        n2194 = Wait (ms)(milliseconds to wait=u32 50) -> ()  [unwired: 1 out]
                      }
                      frame #5 {
                        n2195 = local read "FILE"() -> (w3248:string)
                        n2196 = Concatenate Strings("File Name :" ("Content"), w3248) -> (w3249:string)
                        n2197 = local read "EVENT LOG"() -> (w3252:string)
                        n2198 = call "Event Log.vi"("Content"=w3249, "EVENT LOG"=w3252) -> ("EVENT LOG"=w3251:string)  [unwired: 8 in, 1 out]
                        n2199 = local write "EVENT LOG"(w3251) -> ()
                      }
                      frame #6 {
                        n2200 = Wait (ms)(milliseconds to wait=u32 50) -> ()  [unwired: 1 out]
                      }
                      frame #7 {
                        n2201 = local read "Batch Ref Num :"() -> (w3254:string)
                        n2202 = Concatenate Strings("Batch Ref No :" ("Content"), w3254) -> (w3255:string)
                        n2203 = local read "EVENT LOG"() -> (w3258:string)
                        n2204 = call "Event Log.vi"("Content"=w3255, "EVENT LOG"=w3258) -> ("EVENT LOG"=w3257:string)  [unwired: 8 in, 1 out]
                        n2205 = local write "EVENT LOG"(w3257) -> ()
                      }
                      frame #8 {
                        n2206 = Wait (ms)(milliseconds to wait=u32 50) -> ()  [unwired: 1 out]
                      }
                      frame #9 {
                        n2207 = local read "tested by"() -> (w3260:string)
                        n2208 = Concatenate Strings("Tested By :" ("Content"), w3260) -> (w3261:string)
                        n2209 = local read "EVENT LOG"() -> (w3264:string)
                        n2210 = call "Event Log.vi"("Content"=w3261, "EVENT LOG"=w3264) -> ("EVENT LOG"=w3263:string)  [unwired: 8 in, 1 out]
                        n2211 = local write "EVENT LOG"(w3263) -> ()
                      }
                      frame #10 {
                        n2212 = Wait (ms)(milliseconds to wait=u32 50) -> ()  [unwired: 1 out]
                      }
                      frame #11 {
                        n2213 = local read "TEST STANDARD"() -> (w3267:T3)
                        n2214 = case shown="\"ASTM D6079\", Default" w3267 {
                          tunnel: ["ASTM D6079" "ISO 12156" "CEC F-096-A-06" "Custom"] -> w3266
                          frame "ASTM D6079", Default {
                          }
                          frame "ISO 12156" {
                          }
                          frame "CEC F-096-A-06" {
                          }
                          frame "Custom" {
                          }
                        }
                        n2215 = Concatenate Strings("Test Standard :" ("Content"), w3266) -> (w3268:string)
                        n2216 = local read "EVENT LOG"() -> (w3271:string)
                        n2217 = call "Event Log.vi"("Content"=w3268, "EVENT LOG"=w3271) -> ("EVENT LOG"=w3270:string)  [unwired: 8 in, 1 out]
                        n2218 = local write "EVENT LOG"(w3270) -> ()
                      }
                      frame #12 {
                        n2219 = Wait (ms)(milliseconds to wait=u32 50) -> ()  [unwired: 1 out]
                      }
                      frame #13 {
                        n2220 = local read "Fuel Discription :"() -> (w3277:string)
                        n2221 = Concatenate Strings("Fuel Description :" ("Content"), w3277) -> (w3278:string)
                        n2222 = local read "EVENT LOG"() -> (w3281:string)
                        n2223 = call "Event Log.vi"("Content"=w3278, "EVENT LOG"=w3281) -> ("EVENT LOG"=w3280:string)  [unwired: 8 in, 1 out]
                        n2224 = local write "EVENT LOG"(w3280) -> ()
                      }
                      frame #14 {
                        n2225 = Wait (ms)(milliseconds to wait=u32 50) -> ()  [unwired: 1 out]
                      }
                      frame #15 {
                        n2226 = local read "Remarks :"() -> (w3283:string)
                        n2227 = Concatenate Strings("Remarks :" ("Content"), w3283) -> (w3284:string)
                        n2228 = local read "EVENT LOG"() -> (w3287:string)
                        n2229 = call "Event Log.vi"("Content"=w3284, "EVENT LOG"=w3287) -> ("EVENT LOG"=w3286:string)  [unwired: 8 in, 1 out]
                        n2230 = local write "EVENT LOG"(w3286) -> ()
                      }
                      frame #16 {
                        n2231 = Wait (ms)(milliseconds to wait=u32 50) -> ()  [unwired: 1 out]
                      }
                      frame #17 {
                        n2232 = local read "Operator ID"() -> (w3289:string)
                        n2233 = Concatenate Strings("Operator ID :" ("Content"), w3289) -> (w3291:string)
                        n2234 = local read "EVENT LOG"() -> (w3293:string)
                        n2235 = call "Event Log.vi"("Content"=w3291, "EVENT LOG"=w3293) -> ("EVENT LOG"=w3292:string)  [unwired: 8 in, 1 out]
                        n2236 = local write "EVENT LOG"(w3292) -> ()
                      }
                      frame #18 {
                        n2237 = Wait (ms)(milliseconds to wait=u32 50) -> ()  [unwired: 1 out]
                      }
                      frame #19 {
                        n2238 = disable-structure shown="Disabled" {
                          frame Disabled {
                            n2239 = local read "EVENT LOG"() -> (w3297:string)
                            n2240 = call "Event Log.vi"("Content"="Test Parameter", "EVENT LOG"=w3297) -> ("EVENT LOG"=w3296:string)  [unwired: 8 in, 1 out]
                            n2241 = local write "EVENT LOG"(w3296) -> ()
                          }
                          frame Enabled {
                          }
                        }
                      }
                      frame #20 {
                        n2242 = Wait (ms)(milliseconds to wait=u32 50) -> ()  [unwired: 1 out]
                      }
                      frame #21 {
                        n2243 = local read "Set Hz"() -> (w3301:dbl)
                        n2244 = Number To Fractional String(number=w3301, precision (6)=i16 2) -> (F-format string=w3300:string)  [unwired: 2 in]
                        n2245 = Concatenate Strings("Set Frequency [Hz] :" ("Content"), w3300) -> (w3303:string)
                        n2246 = local read "EVENT LOG"() -> (w3305:string)
                        n2247 = call "Event Log.vi"("Content"=w3303, "EVENT LOG"=w3305) -> ("EVENT LOG"=w3304:string)  [unwired: 8 in, 1 out]
                        n2248 = local write "EVENT LOG"(w3304) -> ()
                      }
                      frame #22 {
                        n2249 = Wait (ms)(milliseconds to wait=u32 50) -> ()  [unwired: 1 out]
                      }
                      frame #23 {
                        n2250 = local read "NORMAL LOAD"() -> (w3308:dbl)
                        n2251 = Number To Fractional String(number=w3308, precision (6)=i16 2) -> (F-format string=w3309:string)  [unwired: 2 in]
                        n2252 = Concatenate Strings("Applied Load [grams] :" ("Content"), w3309) -> (w3311:string)
                        n2253 = local read "EVENT LOG"() -> (w3313:string)
                        n2254 = call "Event Log.vi"("Content"=w3311, "EVENT LOG"=w3313) -> ("EVENT LOG"=w3312:string)  [unwired: 8 in, 1 out]
                        n2255 = local write "EVENT LOG"(w3312) -> ()
                      }
                      frame #24 {
                        n2256 = Wait (ms)(milliseconds to wait=u32 50) -> ()  [unwired: 1 out]
                      }
                      frame #25 {
                        n2257 = local read "Set Strk"() -> (w3316:dbl)
                        n2258 = Number To Fractional String(number=w3316, precision (6)=i16 2) -> (F-format string=w3317:string)  [unwired: 2 in]
                        n2259 = Concatenate Strings("Set Stroke [mm] :" ("Content"), w3317) -> (w3319:string)
                        n2260 = local read "EVENT LOG"() -> (w3321:string)
                        n2261 = call "Event Log.vi"("Content"=w3319, "EVENT LOG"=w3321) -> ("EVENT LOG"=w3320:string)  [unwired: 8 in, 1 out]
                        n2262 = local write "EVENT LOG"(w3320) -> ()
                      }
                      frame #26 {
                        n2263 = Wait (ms)(milliseconds to wait=u32 50) -> ()  [unwired: 1 out]
                      }
                      frame #27 {
                        n2264 = local read "Set Temp"() -> (w3324:dbl)
                        n2265 = Number To Fractional String(number=w3324, precision (6)=i16 2) -> (F-format string=w3325:string)  [unwired: 2 in]
                        n2266 = Concatenate Strings("Set Temperature [deg C] :" ("Content"), w3325) -> (w3327:string)
                        n2267 = local read "EVENT LOG"() -> (w3329:string)
                        n2268 = call "Event Log.vi"("Content"=w3327, "EVENT LOG"=w3329) -> ("EVENT LOG"=w3328:string)  [unwired: 8 in, 1 out]
                        n2269 = local write "EVENT LOG"(w3328) -> ()
                      }
                      frame #28 {
                        n2270 = Wait (ms)(milliseconds to wait=u32 50) -> ()  [unwired: 1 out]
                      }
                      frame #29 {
                        n2271 = local read "Set Rh"() -> (w3332:dbl)
                        n2272 = Number To Fractional String(number=w3332, precision (6)=i16 2) -> (F-format string=w3333:string)  [unwired: 2 in]
                        n2273 = Concatenate Strings("Set Humidity [%RH] :" ("Content"), w3333) -> (w3335:string)
                        n2274 = local read "EVENT LOG"() -> (w3337:string)
                        n2275 = call "Event Log.vi"("Content"=w3335, "EVENT LOG"=w3337) -> ("EVENT LOG"=w3336:string)  [unwired: 8 in, 1 out]
                        n2276 = local write "EVENT LOG"(w3336) -> ()
                      }
                      frame #30 {
                        n2277 = Wait (ms)(milliseconds to wait=u32 50) -> ()  [unwired: 1 out]
                      }
                      frame #31 {
                        n2278 = local read "test time"() -> (w3340:dbl)
                        n2279 = Number To Fractional String(number=w3340, precision (6)=i16 1) -> (F-format string=w3341:string)  [unwired: 2 in]
                        n2280 = Concatenate Strings("Test Duration [mins] :" ("Content"), w3341) -> (w3343:string)
                        n2281 = local read "EVENT LOG"() -> (w3345:string)
                        n2282 = call "Event Log.vi"("Content"=w3343, "EVENT LOG"=w3345) -> ("EVENT LOG"=w3344:string)  [unwired: 8 in, 1 out]
                        n2283 = local write "EVENT LOG"(w3344) -> ()
                      }
                      frame #32 {
